vi "_USB_CAN_PARAM_RW_.vi"(10 "write":bool, 11 "param":T1[](array[typedef]) {"ACR0" format="%x"}) -> (3 "param out":T1[](array[typedef]) {"ACR0" format="%x"})   [LabVIEW 2011]
uses:
  Param.ctl
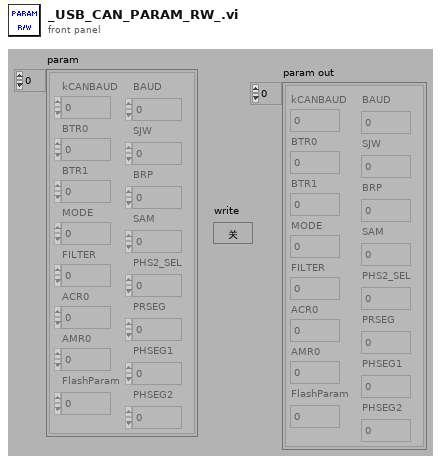
[diagram p1: front panel]
types:
  T1 = typedef "Param.ctl" = cluster{"kCANBAUD":u8, "BTR0":u8, "BTR1":u8, "MODE":u8, "FILTER":u8, "ACR0":u32, "AMR0":u32, "FlashParam":u32, "BAUD":u32, "SJW":u8, "BRP":u8, "SAM":u8, "PHS2_SEL":u8, "PRSEG":u8, "PHSEG1":u8, "PHSEG2":u8}
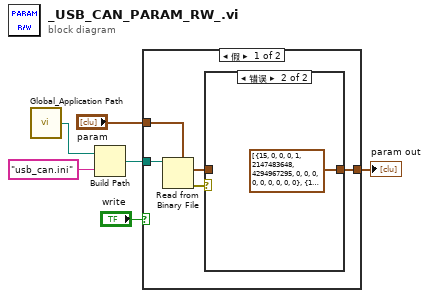
[diagram p0: block diagram]
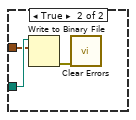
[diagram p3: hidden frame]
diagram:
  n1 = call "Global_Application Path.vi"() -> ("程序路径"=w3:path)  [unwired: 1 in]
  n2 = Build Path(base path=w3, name or relative path="usb_can.ini" ("名称或相对路径")) -> (appended path=w4:path)
  n3 = case shown="假" "write" {
    tunnel: w4 -> [w11 w16]
    tunnel: "param" -> [w10 w15]
    tunnel: [w7 _] -> w2
    frame False {
      n4 = Read from Binary File(5:w10, 11:w11) -> (0:w9:errorcluster, 2:w8:T1[])  [unwired: 4 in, 2 out]
      n5 = case shown="错误" w9 {
        tunnel: [w12 T1[] [{"kCANBAUD"=15, "BTR0"=0, "BTR1"=0, "MODE"=0, "FILTER"=1, "ACR0"=2147483648, "AMR0"=4294967295, "FlashParam"=0, "BAUD"=0, "SJW"=0, "BRP"=0, "SAM"=0, "PHS2_SEL"=0, "PRSEG"=0, "PHSEG1"=0, "PHSEG2"=0}, {"kCANBAUD"=15, "BTR0"=0, "BTR1"=0, "MODE"=0, "FILTER"=1, "ACR0"=2147483648, "AMR0"=4294967295, "FlashParam"=0, "BAUD"=0, "SJW"=0, "BRP"=0, "SAM"=0, "PHS2_SEL"=0, "PRSEG"=0, "PHSEG1"=0, "PHSEG2"=0}] ("param")] -> w7
        tunnel: w8 -> [w12 _]
        frame No Error {
        }
        frame Error {
        }
      }
    }
    frame True {
      n6 = Write to Binary File(file (use dialog)=w16, data=w15) -> (error out=w14:errorcluster)  [unwired: 4 in, 2 out]
      n7 = call <vilib>:"Clear Errors.vi"("error in (no error)"=w14) -> ()  [unwired: 6 in, 1 out]
    }
  }
  "param out" <- w2
